vi "Generate_WayPoints_DIFFERENTPOTONECHLINEWITHPAUSE.vi"(8 "Update Position Loop Wait Time (us)":u32=50000, 11 "Input Cluster":T2={"Scan Rate (um/s)"=15.0, "X Start"=15.0, "X End"=15.0, "Y Start"=15.0, "Y End"=15.0, " Z Start"=15.0, "Number of Lines"=15, "V"=15.0, "Scan Type"=0, "Z End"=15.0, "Approach Rate (um/s)"=15.0, "Squish Approach Rate (um/s)"=15.0, "V 2"=15.0, "HoldTime / us"=15} {"Scan Type" items=["Line Scan (X Major)", "Line Scan (Y Major)"]}) -> (0 "output cluster":T1)   [LabVIEW 2023]
uses:
  TypeDefs/WayPointCluster.ctl
panel:
  in  "WayPointCluster":T1
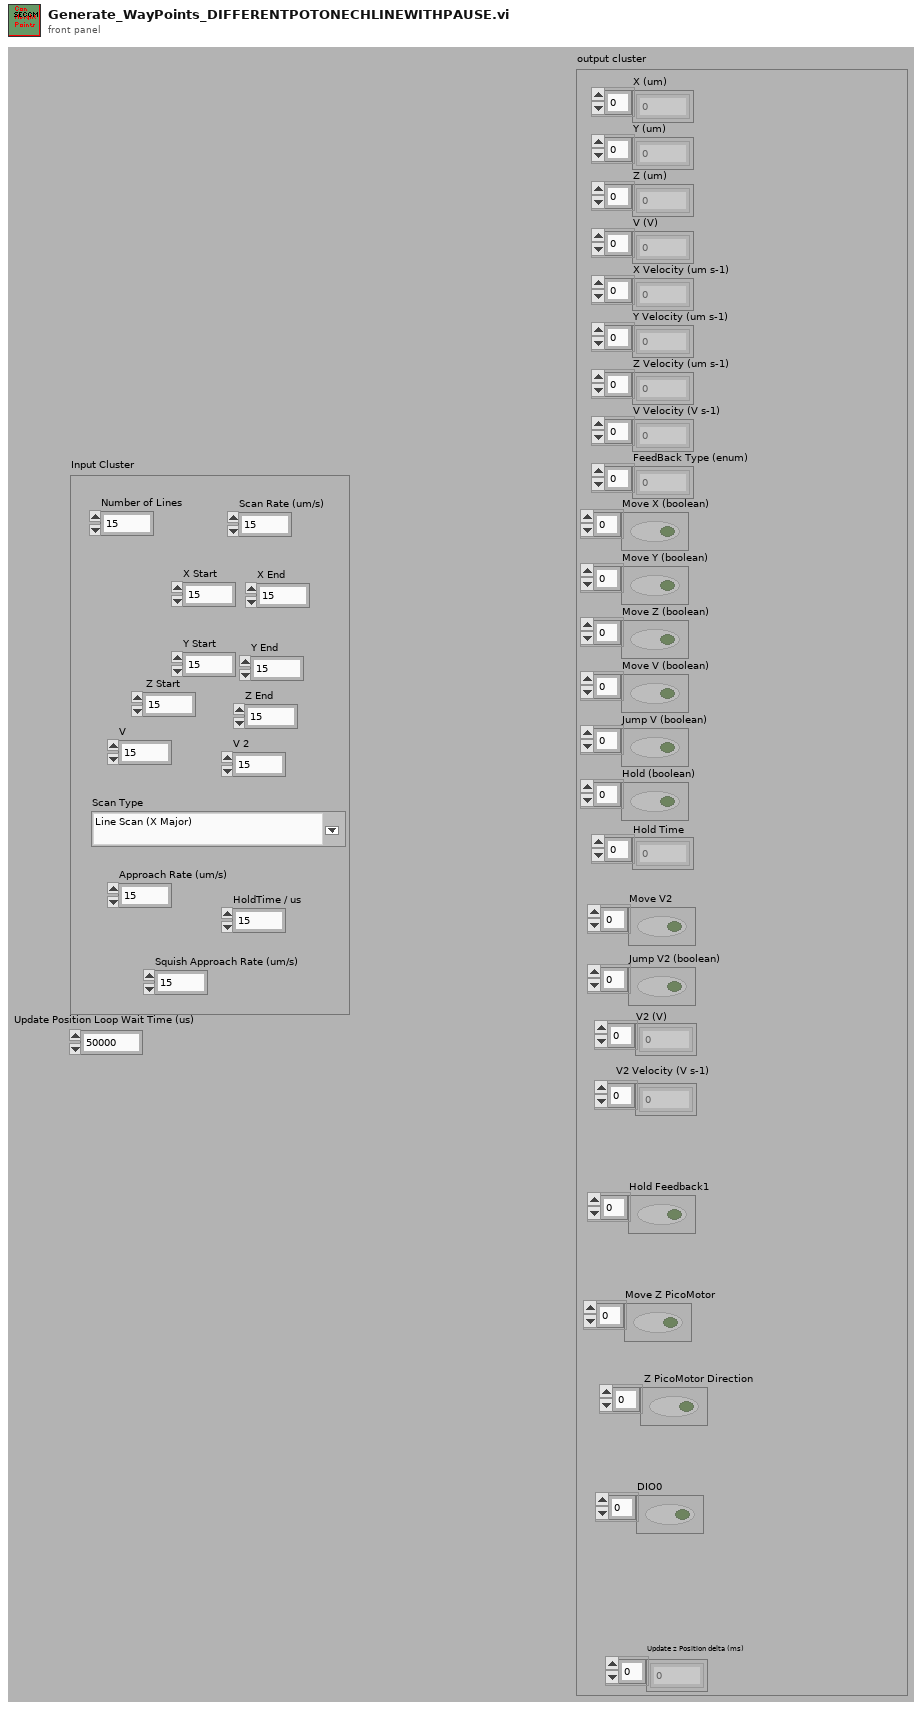
[diagram p1: front panel]
types:
  T1 = typedef "WayPointCluster.ctl" = cluster{"X (um)":dbl[], "Y (um)":dbl[], "Z (um)":dbl[], "V (V)":dbl[], "X Velocity (um s-1)":dbl[], "Y Velocity (um s-1)":dbl[], "Z Velocity (um s-1)":dbl[], "V Velocity (V s-1)":dbl[], "FeedBack Type (enum)":u16[], "Move X (boolean)":bool[], "Move Y (boolean)":bool[], "Move Z (boolean)":bool[], "Move V (boolean)":bool[], "Jump V (boolean)":bool[], "Hold (boolean)":bool[], "Hold Time":u32[], "V2 (V)":dbl[], "Move V2":bool[], "V2 Velocity (V s-1)":dbl[], "Jump V2 (boolean)":bool[], "Update z Position delta (ms)":i16[], "Hold Feedback1":bool[], "Move Z PicoMotor":bool[], " Z PicoMotor Direction":bool[], "DIO0":bool[]}
  T2 = cluster{"Scan Rate (um/s)":dbl, "X Start":dbl, "X End":dbl, "Y Start":dbl, "Y End":dbl, " Z Start":dbl, "Number of Lines":u32, "V":dbl, "Scan Type":u16, "Z End":dbl, "Approach Rate (um/s)":dbl, "Squish Approach Rate (um/s)":dbl, "V 2":dbl, "HoldTime / us":u32}
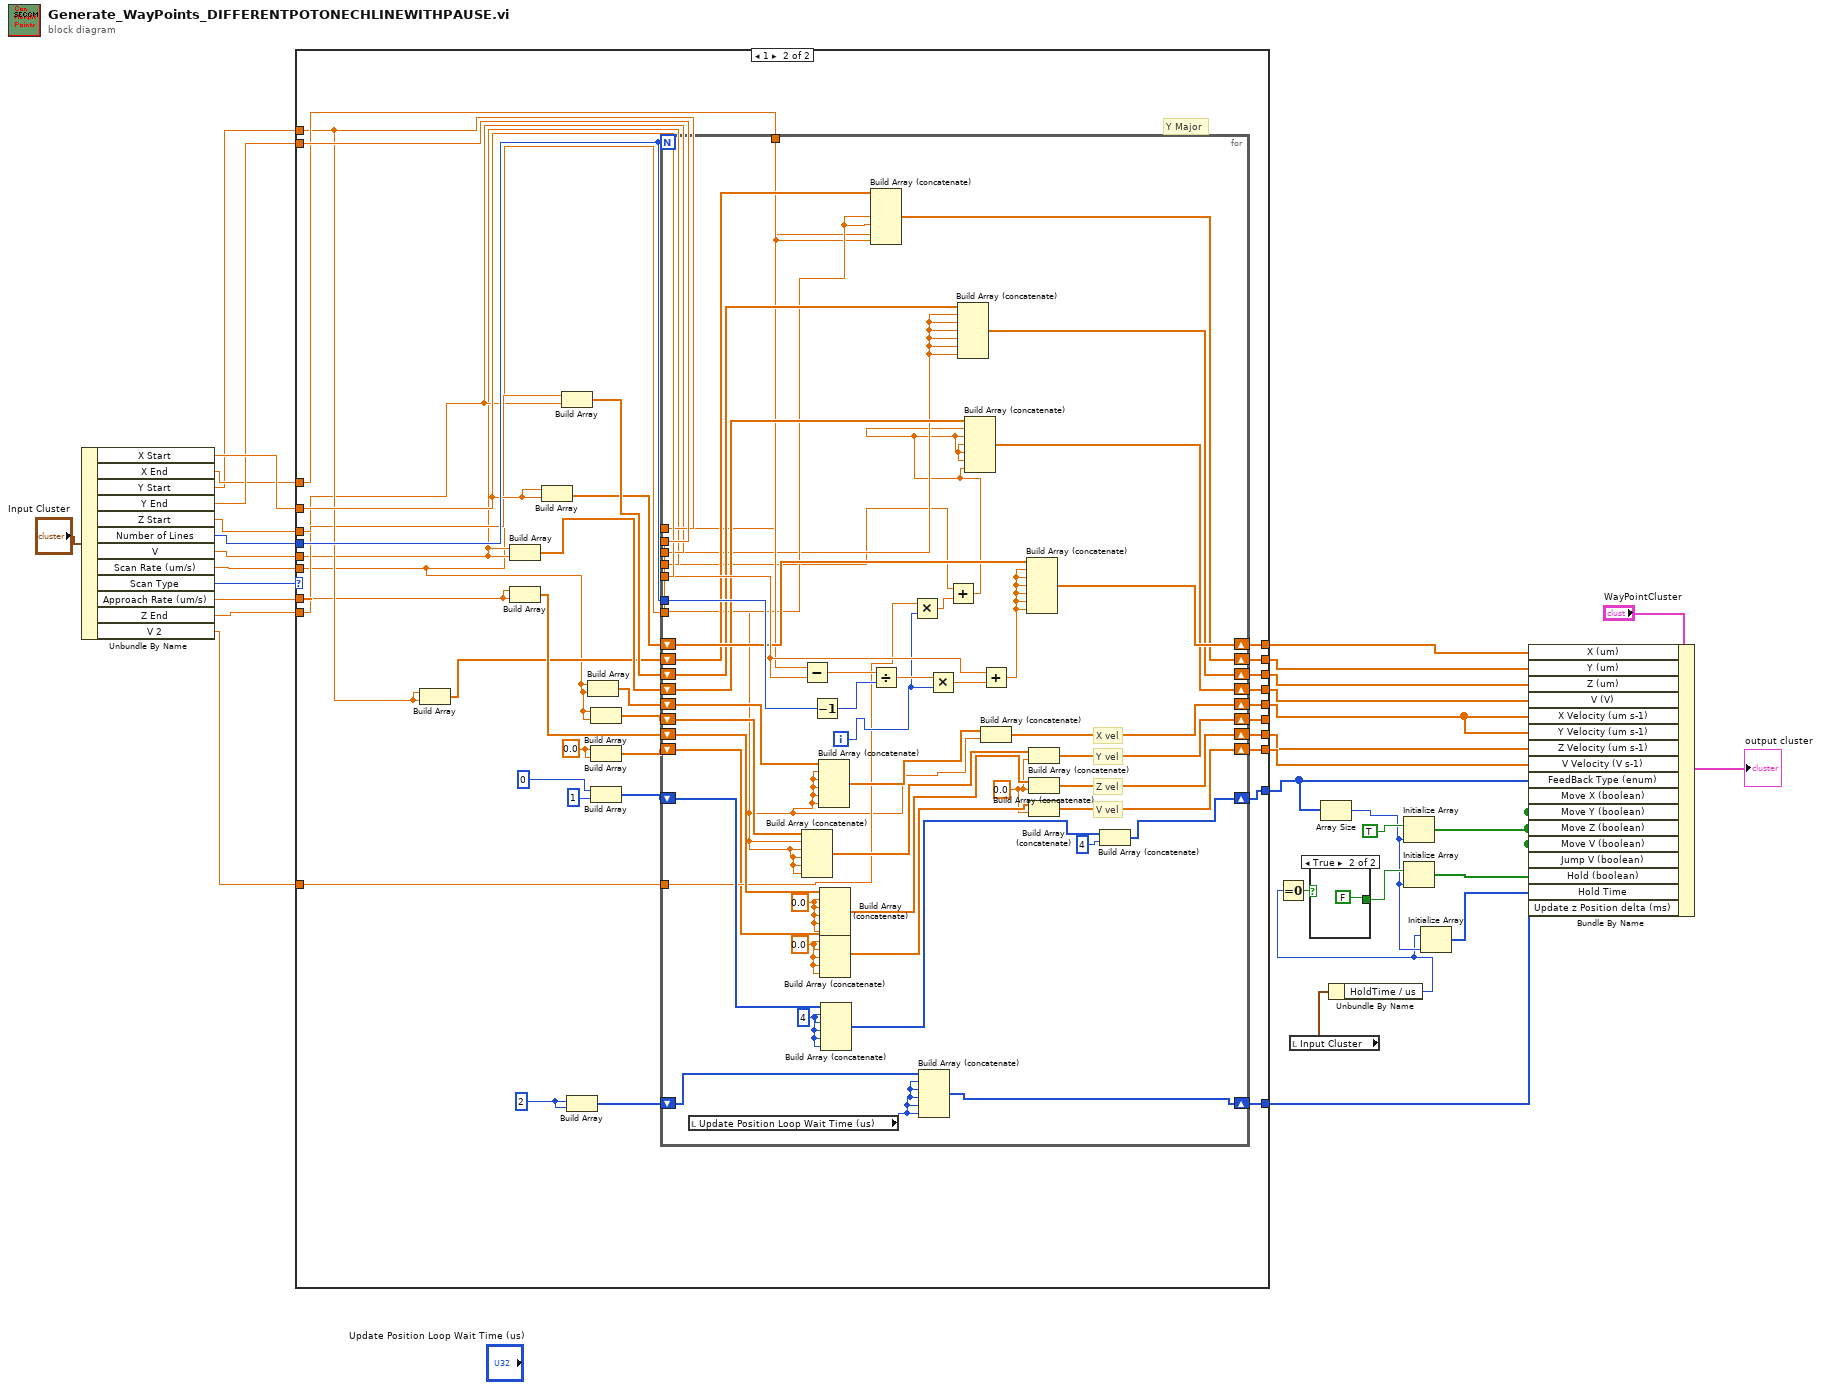
[diagram p0: block diagram]
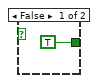
[diagram p2: hidden frame]
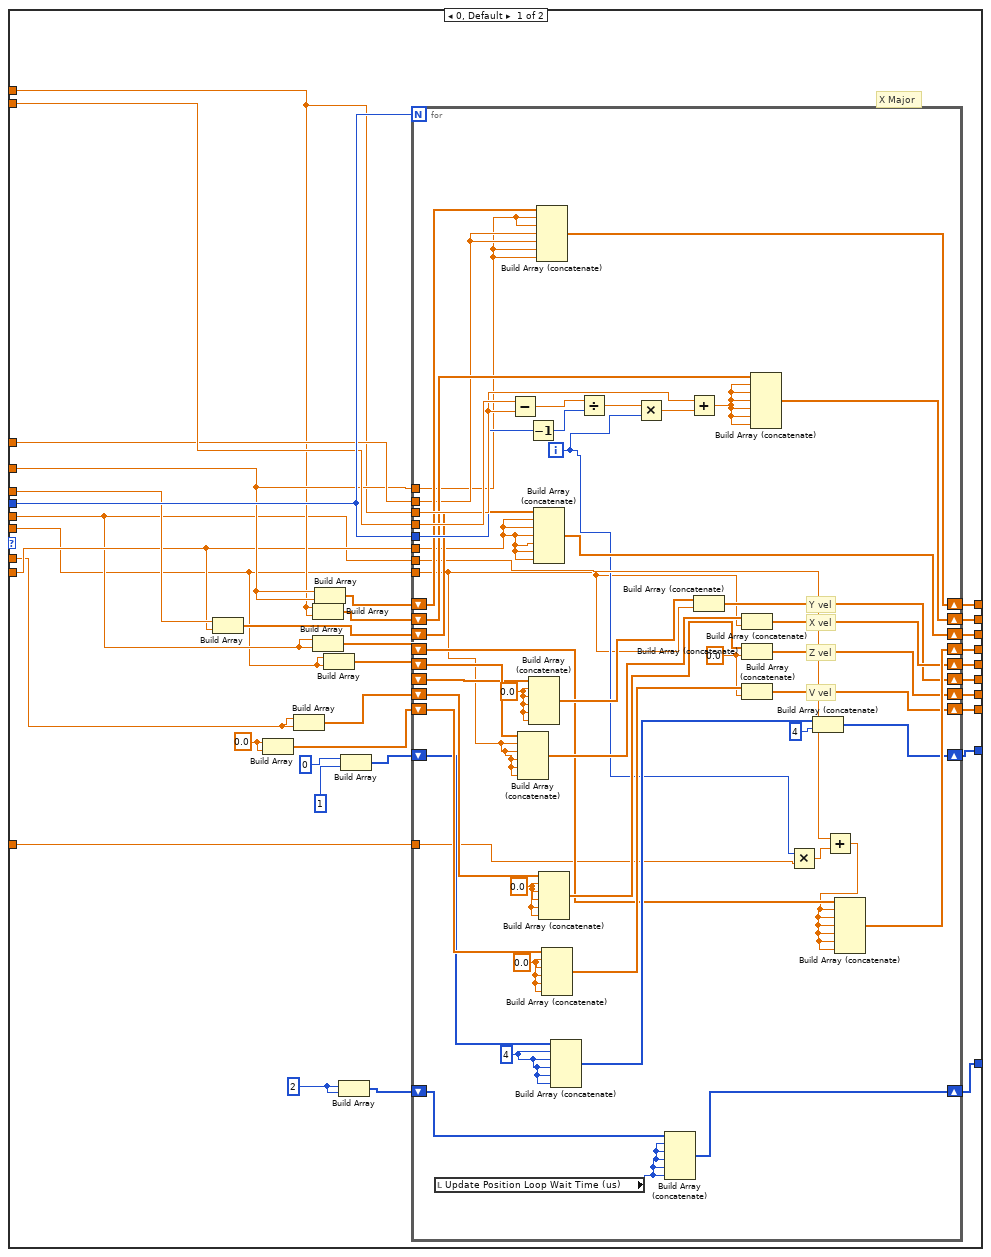
[diagram p3: hidden frame]
diagram:
  n1 = Unbundle By Name("Input Cluster") -> ("X Start"=w31:dbl, "X End"=w17:dbl, "Y Start"=w7:dbl, "Y End"=w27:dbl, "Z Start"=w30:dbl, "Number of Lines"=w29:u32, "V"=w32:dbl, "Scan Rate (um/s)"=w28:dbl, "Scan Type"=w23:u16, "Approach Rate (um/s)"=w19:dbl, "Z End"=w18:dbl, "V 2"=w8:dbl)
  n2 = case shown="1" w23 {
    tunnel: w32 -> [w41 w124]
    tunnel: w31 -> [w45 w128]
    tunnel: w30 -> [w43 w126]
    tunnel: w29 -> [w67 w151]
    tunnel: w28 -> [w40 w122]
    tunnel: w7 -> [w44 w127]
    tunnel: w27 -> [w66 w144]
    tunnel: [w65 w142] -> w6
    tunnel: [w64 w145] -> w22
    tunnel: [w63 w150] -> w20
    tunnel: [w62 w146] -> w26
    tunnel: [w61 w149] -> w21
    tunnel: [w60 w143] -> _
    tunnel: [w59 w148] -> w25
    tunnel: [w58 w147] -> w24
    tunnel: w19 -> [w39 w123]
    tunnel: [w57 w141] -> w15
    tunnel: w18 -> [w42 w125]
    tunnel: w17 -> [w47 w131]
    tunnel: w8 -> [w46 w129]
    tunnel: [w34 w117] -> w4
    frame 0, Default {
      w36 = u32 2 ("element")
      w38 = 0.0 ("element")
      # "X Major"
      n3 = Build Array(w43, w42) -> (w50:dbl[])
      n4 = Build Array(w38, w38) -> (w54:dbl[])
      n5 = Build Array(w39, w39) -> (w53:dbl[])
      n6 = Build Array(w44, w44) -> (w49:dbl[])
      n7 = Build Array(w41, w41) -> (w51:dbl[])
      n8 = Build Array(w45, w45) -> (w48:dbl[])
      n9 = Build Array(w40, w40) -> (w52:dbl[])
      n10 = Build Array(w36, w36) -> (w35:u32[])
      n11 = Build Array(u16 0 ("element"), u16 1 ("element")) -> (w55:u16[])
      n12 = for {
        N: w67 -> [_]
        tunnel: w45 -> [w85]
        tunnel: w47 -> [w86]
        tunnel: w42 -> [w83]
        tunnel: w41 -> [w78]
        tunnel: w44 -> [w115]
        tunnel: w66 -> [w116]
        tunnel: w67 -> [w111]
        tunnel: w40 -> [w71]
        shift-right: [w93] -> w65
        shift-left: w52 -> [w110]
        shift-right: [w101] -> w64
        shift-left: w49 -> [w109]
        shift-right: [w99] -> w63
        shift-left: w51 -> [w87]
        shift-right: [w102] -> w62
        shift-left: w48 -> [w108]
        shift-right: [w100] -> w61
        shift-left: w50 -> [w107]
        shift-right: [w91] -> w60
        shift-left: _ -> [w106]
        shift-right: [w95] -> w58
        shift-left: w53 -> [w105]
        shift-right: [w96] -> w59
        shift-left: w54 -> [w104]
        shift-right: [w88] -> w57
        shift-left: w55 -> [w90]
        tunnel: w46 -> [w76]
        shift-right: [w68] -> w34
        shift-left: w35 -> [w70]
        i -> [w74]
        w73 = 0.0 ("element")
        w79 = u16 4 ("element")
        w81 = 0.0 ("element")
        w82 = 0.0 ("element")
        w80 = 0.0 ("element")
        # "Y vel"
        # "X vel"
        # "Z vel"
        # "V vel"
        n13 = local read "Update Position Loop Wait Time (us)"() -> (w69:u32)
        n14 = Subtract(x=w116, y=w115) -> (x-y=w114:dbl)
        n15 = Build Array (concatenate)(w110, w71, w71, w71, w71, w71) -> (w94:dbl[])
        n16 = Decrement(x=w111) -> (x-1=w103:u32)
        n17 = Build Array (concatenate)(w106, w82, w82, w82, w82, w82) -> (w92:dbl[])
        n18 = Build Array (concatenate)(w107, w83, w83, w83, w83, w83, w83) -> (w100:dbl[])
        n19 = Build Array (concatenate)(w108, w85, w85, w86, w86, w85, w85) -> (w102:dbl[])
        n20 = Build Array (concatenate)(w105, w80, w80, w80, w80, w80) -> (w98:dbl[])
        n21 = Build Array (concatenate)(w104, w81, w81, w81, w81, w81) -> (w97:dbl[])
        n22 = Build Array (concatenate)(w90, w79, w79, w79, w79, w79) -> (w89:u16[])
        n23 = Divide(x=w114, y=w103) -> (x/y=w112:dbl)
        n24 = Multiply(x=w112, y=w74) -> (x*y=w113:dbl)
        n25 = Build Array (concatenate)(w70, w69, w69, w69, w69, w69) -> (w68:u32[])
        n26 = Add(x=w115, y=w113) -> (x+y=w84:dbl)
        n27 = Build Array (concatenate)(w92, w71) -> (w91:dbl[])
        n28 = Build Array (concatenate)(w94, w71) -> (w93:dbl[])
        n29 = Build Array (concatenate)(w98, w73) -> (w95:dbl[])
        n30 = Build Array (concatenate)(w97, w73) -> (w96:dbl[])
        n31 = Build Array (concatenate)(w109, w84, w84, w84, w84, w84, w84) -> (w101:dbl[])
        n32 = Multiply(x=w74, y=w76) -> (x*y=w75:dbl)
        n33 = Build Array (concatenate)(w89, u16 4 ("element")) -> (w88:u16[])
        n34 = Add(x=w78, y=w75) -> (x+y=w77:dbl)
        n35 = Build Array (concatenate)(w87, w77, w77, w77, w77, w77, w77) -> (w99:dbl[])
      }
    }
    frame 1 {
      w119 = u16 2 ("element")
      w121 = 0.0 ("element")
      # "Y Major"
      n36 = Build Array(w127, w127) -> (w130:dbl[])
      n37 = Build Array(w124, w124) -> (w134:dbl[])
      n38 = Build Array(w123, w123) -> (w137:dbl[])
      n39 = Build Array(w128, w128) -> (w132:dbl[])
      n40 = Build Array(w126, w125) -> (w133:dbl[])
      n41 = Build Array(w119, w119) -> (w118:u16[])
      n42 = Build Array(w122, w122) -> (w135:dbl[])
      n43 = Build Array(w122, w122) -> (w136:dbl[])
      n44 = Build Array(w121, w121) -> (w140:dbl[])
      n45 = Build Array(u16 0 ("element"), u16 1 ("element")) -> (w138:u16[])
      n46 = for {
        N: w151 -> [_]
        tunnel: w127 -> [w169]
        tunnel: w144 -> [w170]
        tunnel: w125 -> [w168]
        tunnel: w124 -> [w160]
        tunnel: w128 -> [w199]
        tunnel: w151 -> [w195]
        tunnel: w122 -> [w156]
        shift-right: [w185] -> w142
        shift-left: w135 -> [w184]
        shift-right: [w179] -> w146
        shift-left: w132 -> [w194]
        shift-right: [w176] -> w150
        shift-left: w134 -> [w193]
        shift-right: [w178] -> w145
        shift-left: w130 -> [w192]
        shift-right: [w177] -> w149
        shift-left: w133 -> [w191]
        shift-right: [w186] -> w143
        shift-left: w136 -> [w183]
        shift-right: [w188] -> w147
        shift-left: w137 -> [w190]
        shift-right: [w189] -> w148
        shift-left: w140 -> [w155]
        shift-right: [w172] -> w141
        shift-left: w138 -> [w174]
        tunnel: w131 -> [w171]
        tunnel: w129 -> [w161]
        shift-right: [w152] -> w117
        shift-left: w118 -> [w154]
        i -> [w162]
        w158 = 0.0 ("element")
        w166 = u16 4 ("element")
        w165 = 0.0 ("element")
        w164 = 0.0 ("element")
        # "Y vel"
        # "X vel"
        # "Z vel"
        # "V vel"
        n47 = local read "Update Position Loop Wait Time (us)"() -> (w153:u32)
        n48 = Subtract(x=w171, y=w199) -> (x-y=w198:dbl)
        n49 = Build Array (concatenate)(w183, w156, w156, w156, w156, w156) -> (w181:dbl[])
        n50 = Decrement(x=w195) -> (x-1=w187:u32)
        n51 = Build Array (concatenate)(w184, w156, w156, w156, w156, w156) -> (w180:dbl[])
        n52 = Build Array (concatenate)(w190, w164, w164, w164, w164, w164) -> (w175:dbl[])
        n53 = Build Array (concatenate)(w155, w165, w165, w165, w165, w165) -> (w182:dbl[])
        n54 = Build Array (concatenate)(w174, w166, w166, w166, w166, w166) -> (w173:u16[])
        n55 = Build Array (concatenate)(w192, w169, w169, w170, w170, w169, w169) -> (w178:dbl[])
        n56 = Divide(x=w198, y=w187) -> (x/y=w196:dbl)
        n57 = Multiply(x=w161, y=w162) -> (x*y=w163:dbl)
        n58 = Build Array (concatenate)(w154, w153, w153, w153, w153, w153) -> (w152:u32[])
        n59 = Multiply(x=w196, y=w162) -> (x*y=w197:dbl)
        n60 = Add(x=w160, y=w163) -> (x+y=w159:dbl)
        n61 = Build Array (concatenate)(w191, w168, w168, w168, w168, w168, w168) -> (w177:dbl[])
        n62 = Build Array (concatenate)(w193, w159, w159, w159, w159, w159, w159) -> (w176:dbl[])
        n63 = Add(x=w199, y=w197) -> (x+y=w167:dbl)
        n64 = Build Array (concatenate)(w180, w156) -> (w185:dbl[])
        n65 = Build Array (concatenate)(w194, w167, w167, w167, w167, w167, w167) -> (w179:dbl[])
        n66 = Build Array (concatenate)(w181, w158) -> (w186:dbl[])
        n67 = Build Array (concatenate)(w175, w158) -> (w188:dbl[])
        n68 = Build Array (concatenate)(w182, w158) -> (w189:dbl[])
        n69 = Build Array (concatenate)(w173, u16 4 ("element")) -> (w172:u16[])
      }
    }
  }
  n70 = local read "Input Cluster"() -> (w10:T2)
  n71 = Array Size(array=w15) -> (size(s)=w11:i32)
  n72 = Unbundle By Name(w10) -> ("HoldTime / us"=w2:u32)
  n73 = Equal To 0?(x=w2) -> (x = 0?=w3:bool)
  n74 = case shown="True" w3 {
    tunnel: [TRUE FALSE] -> w13
    frame False {
    }
    frame True {
    }
  }
  n75 = Initialize Array(TRUE, w11) -> (w14:bool[])
  n76 = Initialize Array(w13, w11) -> (w12:bool[])
  n77 = Initialize Array(w2, w11) -> (w9:u32[])
  n78 = Bundle By Name(cluster="WayPointCluster", "X (um)"=w26, "Y (um)"=w22, "Z (um)"=w21, "V (V)"=w20, "X Velocity (um s-1)"=w6, "Y Velocity (um s-1)"=w6, "Z Velocity (um s-1)"=w24, "V Velocity (V s-1)"=w25, "FeedBack Type (enum)"=w15, "Move X (boolean)"=w14, "Move Y (boolean)"=w14, "Move Z (boolean)"=w14, "Move V (boolean)"=w14, "Jump V (boolean)"=w14, "Hold (boolean)"=w12, "Hold Time"=w9, "Update z Position delta (ms)"=w4) -> (→"output cluster":T1)
